vi "ConfigDlg.vi"(8 "error in (no error)":errorcluster, 11 "CorrFactor in":refnum<class "CorrFactor.lvclass">) -> (0 "error out":errorcluster, 2 "Changed":bool, 3 "CorrFactor out":refnum<class "CorrFactor.lvclass">)   [LabVIEW 2018, in "AnalysisPlugins.lvlib" / "CorrFactor.lvclass"]
uses:
  CorrFactor.lvclass
  Typedefs/3458 Params.ctl
  Typedefs/clAnalysisConfig.ctl
  <vilib>/Utility/config.llb/NI_LVConfig.lvlib
panel:
  in  "FunctionIniFilePath":path caption="Test Function .ini File"
  in  "btnSaveAs":bool
  in  "btnFuncConfig":bool
  in  "BtnCancel":bool
  in  "btnSave":bool
  in  "clAnalysisConfig":T1={"HP 3458 address"="", "3458  Params:"={"Record Size"=4096, "Input Freq (Hz)"=50.0, "# Cycles (Desired)"=501.0, "Sampling Mode:"=1, "# of Record Avgs./Meas."=1, "Trigger Mode"=0, "Trig. Level (%)"=0.0, "# of Meas. Runs"=5, "Trigger Slope"=0}} {"3458  Params:"."Sampling Mode:" items=["DCV", "DCV (Corrected)", "DSDC", "SSDC"]; "3458  Params:"."Trigger Mode" items=["LEVEL", "EXTERNAL"]; "3458  Params:"."Trigger Slope" items=["POSITIVE", "NEGATIVE"]}
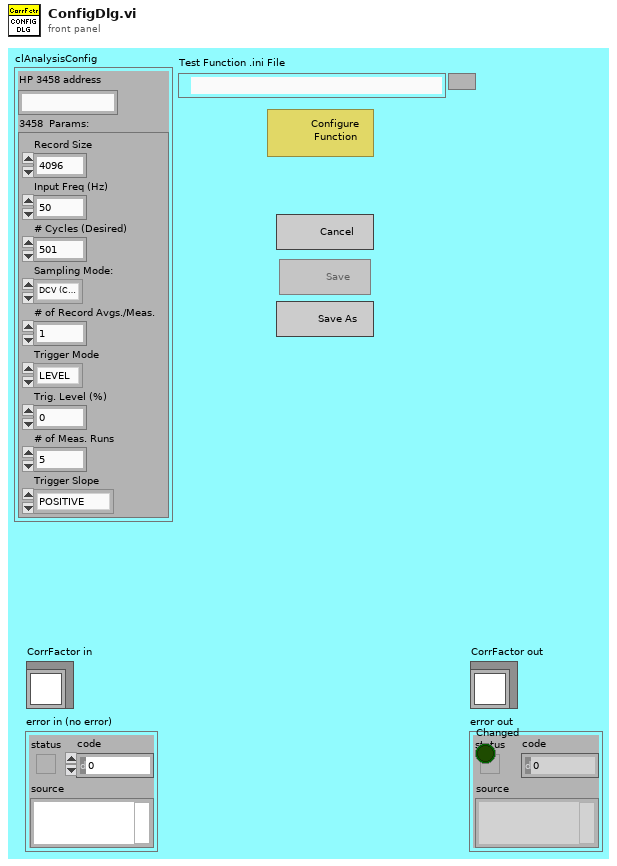
[diagram p1: front panel]
types:
  T1 = typedef "AnalysisPlugins.lvlib/CorrFactor.lvclass/clAnalysisConfig.ctl" = cluster{"HP 3458 address":string, "3458  Params:":T2}
  T2 = typedef "AnalysisPlugins.lvlib/CorrFactor.lvclass/3458 Params.ctl" = cluster{"Record Size":i32, "Input Freq (Hz)":dbl, "# Cycles (Desired)":dbl, "Sampling Mode:":u16, "# of Record Avgs./Meas.":i32, "Trigger Mode":u16, "Trig. Level (%)":dbl, "# of Meas. Runs":i32, "Trigger Slope":u16}
  T3 = enum8{"Enabled", "Disabled", "Disabled and Grayed Out"}
  T4 = enum32{"Invalid", "Default", "Floating", "Floating/Auto-Hide", "Modal"}
  T5 = typedef "NI_LVConfig.lvlib/Config Data RefNum.ctl" = refnum<k1>
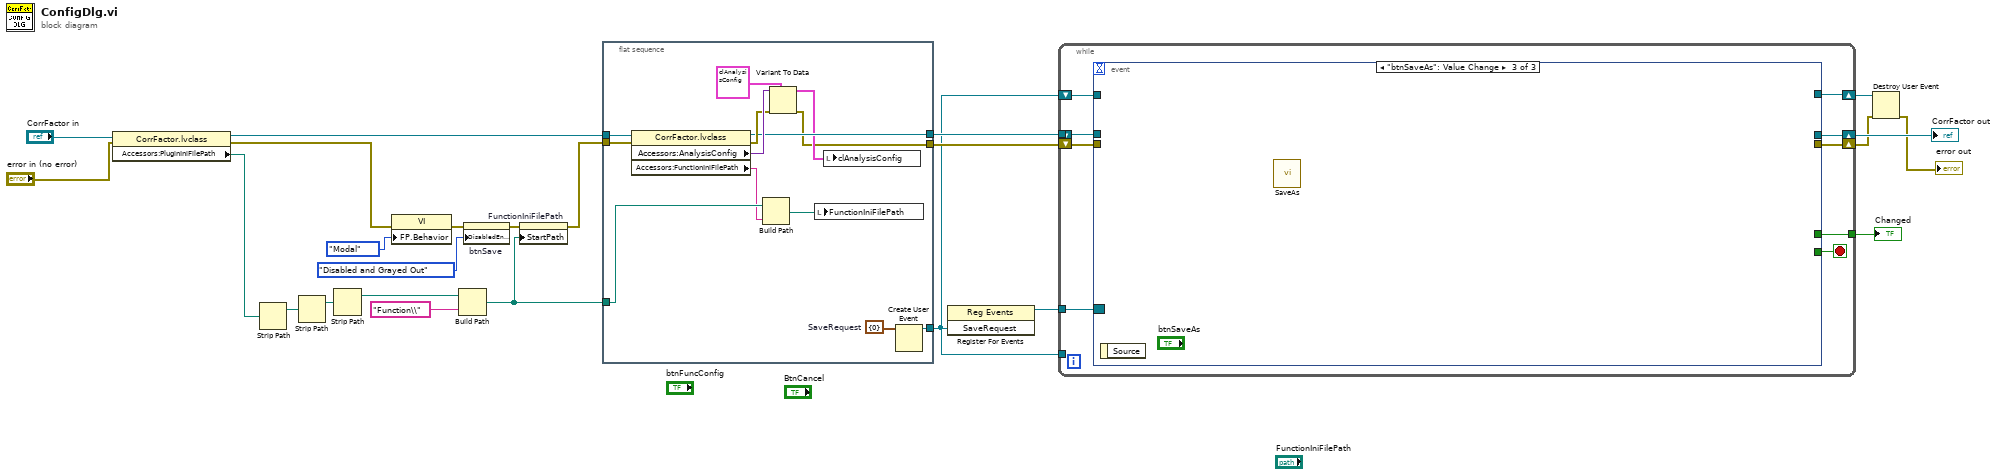
[diagram p0: block diagram]
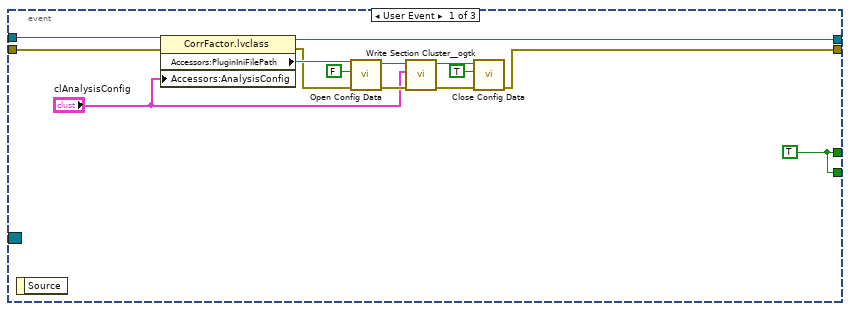
[diagram p2: hidden frame]
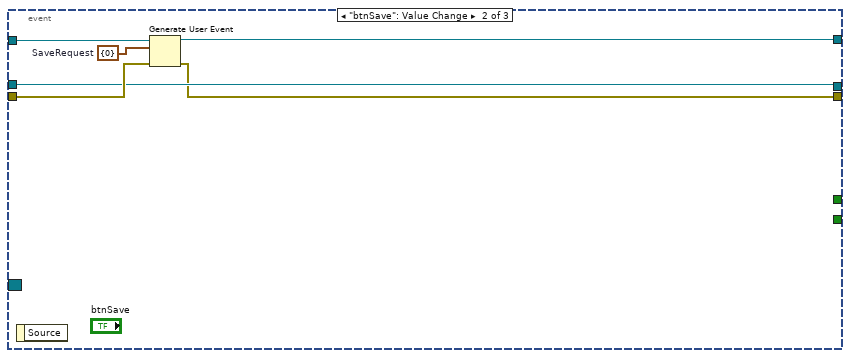
[diagram p3: hidden frame]
diagram:
  n1 = property class="CorrFactor.lvclass"(reference="CorrFactor in", error in="error in (no error)") -> (reference out=w12:refnum<class "CorrFactor.lvclass">, error out=w14:errorcluster, "Accessors:PluginIniFilePath"=w13:path)
  n2 = Strip Path(path=w13) -> (stripped path=w17:path)  [unwired: 1 out]
  n3 = Strip Path(path=w17) -> (stripped path=w16:path)  [unwired: 1 out]
  n4 = Strip Path(path=w16) -> (stripped path=w15:path)  [unwired: 1 out]
  n5 = property class="VI"(error in=w14, "FP.Behavior"=T4."Modal" ("Front Panel Window:Behavior")) -> (error out=w21:errorcluster)  [unwired: 1 in, 1 out]
  n6 = Build Path(base path=w15, name or relative path="Function\\") -> (appended path=w10:path)
  n7 = property on="btnSave" class="Bool"(error in=w21, "DisabledEnum"=T3."Disabled and Grayed Out" ("Disabled")) -> (error out=w19:errorcluster)  [unwired: 1 in, 1 out]
  n8 = property on="FunctionIniFilePath" class="Path"(error in=w19, "StartPath"=w10) -> (error out=w11:errorcluster)  [unwired: 1 in, 1 out]
  n9 = flat-sequence {
    tunnel: w12 -> [w37]
    tunnel: w11 -> [w36]
    tunnel: w10 -> [w32]
    tunnel: [w29] -> w8
    tunnel: [w27] -> w7
    tunnel: [w25] -> w6
    frame #0 {
      w30 = cluster{"Num":i32} {"Num"=0}  # SaveRequest
      n10 = property class="CorrFactor.lvclass"(reference=w37, error in=w36) -> (reference out=w29:refnum<class "CorrFactor.lvclass">, error out=w33:errorcluster, "Accessors:AnalysisConfig"=w34:variant, "Accessors:FunctionIniFilePath"=w31:string)
      n11 = Build Path(base path=w32, name or relative path=w31) -> (appended path=w26:path)
      n12 = Variant To Data(error in=w33, type=T1 {"HP 3458 address"="", "3458  Params:"={"Record Size"=4096, "Input Freq (Hz)"=50.0, "# Cycles (Desired)"=501.0, "Sampling Mode:"=1, "# of Record Avgs./Meas."=1, "Trigger Mode"=0, "Trig. Level (%)"=0.0, "# of Meas. Runs"=5, "Trigger Slope"=0}} ("clAnalysisConfig"), Variant=w34) -> (data=w28:T1, error out=w27:errorcluster)
      n13 = local write "FunctionIniFilePath"(w26) -> ()
      n14 = local write "clAnalysisConfig"(w28) -> ()
      n15 = Create User Event(user event datatype=w30) -> (user event=w25:refnum<user-event>)  [unwired: 1 in, 1 out]
    }
  }
  n16 = register-events(w6) -> (reference out=w9:refnum<event-registration>)  [unwired: 2 in, 1 out]
  n17 = while {
    tunnel: w6 -> [_]
    tunnel: w9 -> [w46]
    tunnel: w8 -> [w45]
    shift-right: [w40] -> w4
    shift-left: w6 -> [w43]
    shift-right: [w42] -> w5
    shift-left: _ -> [_]
    shift-right: [w41] -> w3
    shift-left: w7 -> [w44]
    tunnel: [w39] -> w1
    stop <- w38 stop-if-true
    n18 = event shown="[2] \"btnSaveAs\": Value Change" {
      selector: w46 -> [_ _ _]
      dyn-events: _ -> [_ _ _]
      timeout: _ -> [_ _ _]
      tunnel: w45 -> [w60 w63 _]
      tunnel: w44 -> [w59 w64 _]
      tunnel: w43 -> [_ w66 _]
      tunnel: [w49 w63 _] -> w42
      tunnel: [w48 w61 _] -> w41
      tunnel: [_ w62 _] -> w40
      tunnel: [w47 _ _] -> w39
      tunnel: [w47 _ _] -> w38
      event User Event {
        w47 = TRUE
        n19 = event-data() -> ()  [unwired: 1 in, 1 out]
        n20 = property class="CorrFactor.lvclass"(reference=w60, error in=w59, "Accessors:AnalysisConfig"="clAnalysisConfig") -> (reference out=w49:refnum<class "CorrFactor.lvclass">, error out=w56:errorcluster, "Accessors:PluginIniFilePath"=w58:path)
        n21 = call <vilib>:"Open Config Data.vi"("error in (no error)"=w56, "create file if necessary (T)"=FALSE, "configuration file path"=w58) -> ("error out"=w55:errorcluster, "refnum"=w54:T5)  [unwired: 6 in, 1 out]
        n22 = call <userlib>:"Write Section Cluster__ogtk.vi"("error in (no error)"=w55, "Section Formatted Cluster"="clAnalysisConfig", "refnum"=w54) -> ("error out"=w52:errorcluster, "dup refnum"=w51:T5)  [unwired: 7 in]
        n23 = call <vilib>:"Close Config Data.vi"("error in (no error)"=w52, "write file if changed (T)"=TRUE, "refnum"=w51) -> ("error out"=w48:errorcluster)  [unwired: 7 in, 1 out]
      }
      event "btnSave": Value Change {
        w65 = cluster{"Num":i32} {"Num"=0}  # SaveRequest
        n24 = event-data() -> ()  [unwired: 1 in, 1 out]
        n25 = Generate User Event(user event=w66, event data cluster=w65, error in=w64) -> (user event out=w62:refnum<user-event>, error out=w61:errorcluster)  [unwired: 1 in]
      }
      event "btnSaveAs": Value Change {
        n26 = event-data() -> ()  [unwired: 1 in, 1 out]
        n27 = call "SaveAs.vi"() -> ()  [unwired: 11 in, 1 out]
      }
    }
  }
  "CorrFactor out" <- w5
  "Changed" <- w1
  n28 = Destroy User Event(user event=w4, error in=w3) -> (error out=→"error out":errorcluster)
